vi "MessageDialog.vi"(8 "error in (no error)":errorcluster, 11 "Message":string) -> (0 "error out":errorcluster)   [LabVIEW 2019]
panel:
  in  "OK":bool
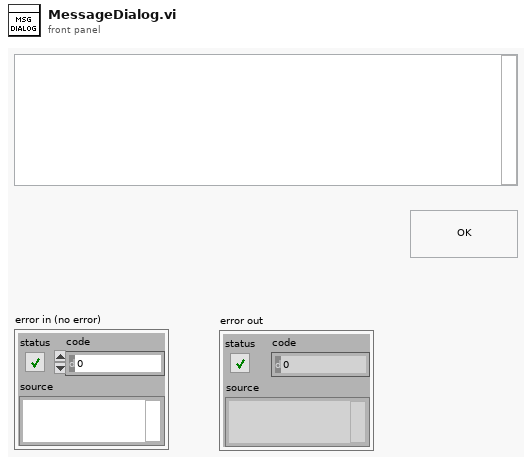
[diagram p1: front panel]
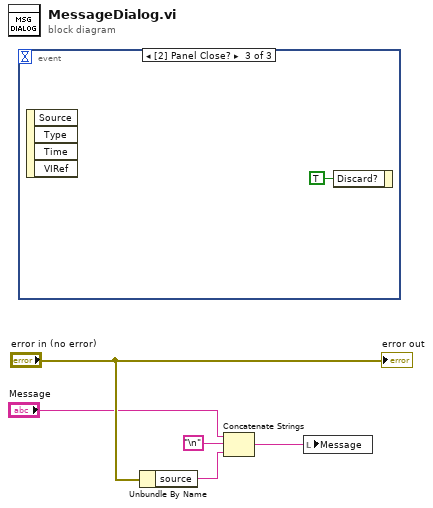
[diagram p0: block diagram]
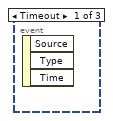
[diagram p2: hidden frame]
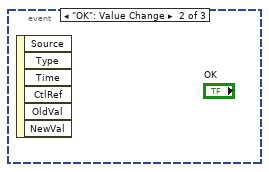
[diagram p3: hidden frame]
diagram:
  n1 = event shown="[2] Panel Close?" {
    selector: _ -> [_ _ _]
    dyn-events: _ -> [_ _ _]
    timeout: _ -> [_ _ _]
    event Timeout {
      n2 = event-data() -> ()  [unwired: 1 in, 3 out]
    }
    event "OK": Value Change {
      n3 = event-data() -> ()  [unwired: 1 in, 6 out]
    }
    event Panel Close? {
      n4 = event-data() -> ()  [unwired: 1 in, 4 out]
      n5 = event-data("Discard?"=TRUE) -> ()  [unwired: 1 in, 1 out]
    }
  }
  n6 = Unbundle By Name("error in (no error)") -> ("source"=w1:string)
  n7 = Concatenate Strings("Message", "\n", w1) -> (w2:string)
  n8 = local write "Message"(w2) -> ()
  "error out" <- "error in (no error)"
